vi "Airflow 05.03.16.vi"(0 "Helium":refnum<vi>, 1 "Write refnum In":refnum<file>, 3 "Stop in":refnum<vi>, 5 "Nitrogen":refnum<vi>, 9 "Chemical":refnum<vi>, 11 "Vacuum":refnum<vi>, 12 "Error in":errorcluster, 13 "Boolean":bool, 14 "String out":refnum<vi>) -> (4 "refnum out 2":refnum<file>, 6 "error out":errorcluster, 10 "VISA resource name out":refnum<visa-resource-name>, 15 "Error out VISA":errorcluster)   [LabVIEW 2017]
uses:
  <vilib>/Platform/TimedLoop/XDataNode/timing_clust.ctl
  <vilib>/Platform/TimedLoop/XDataNode/nitl_modes.ctl
  <vilib>/Platform/TimedLoop/XDataNode/wakeup.ctl
  <vilib>/Instr/_visa.llb/VISA Configure Serial Port (Instr).vi
  <vilib>/Utility/file.llb/Read Delimited Spreadsheet (DBL).vi
  <vilib>/platform/TimedLoop/XDataNode/XDataNode.xnode
  <vilib>/Platform/TimedLoop/XDataNode/XDNodeRunTimeDep.lvlib
panel:
  out "Value":dbl
  out "element":dbl
  in  "Vacuum 2":dbl
  out "concatenated string":string
  # "© The Regents of the University of California, Davis campus, 2019. This material is available as open source for research and personal use under a Creative Commons Attribution-NonCommercial-NoDerivatives 4.0 International Public License (https://creativecommons.org/licenses/by-nc-nd/4.0/)."
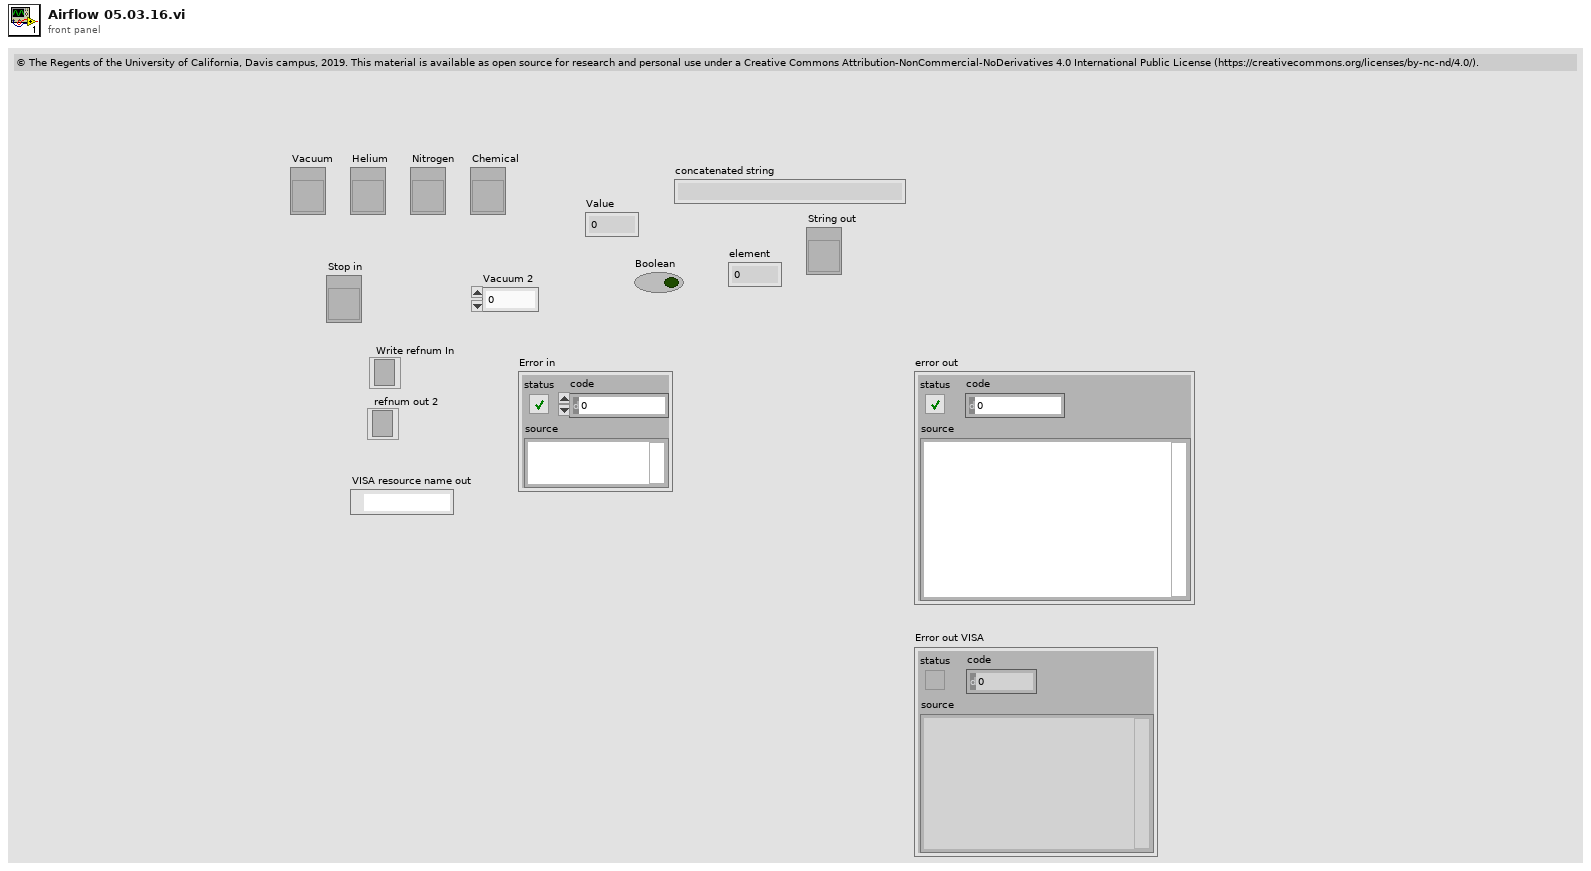
[diagram p1: front panel]
types:
  T1 = typedef "XDNodeRunTimeDep.lvlib/timing_clust.ctl" = cluster{"Expected End [f-1]":u64, "Actual End [f-1]":u64, "Finished Late? [f-1]":bool, "Expected End [i-1]":u64, "Actual End [i-1]":u64, "Finished Late? [i-1]":bool, "Expected Start [i]":u64, "Actual Start [i]":u64, "Expected Start [f]":u64, "Actual Start [f]":u64, "Source Name":string, "Structure Name":string, "Period":i64, "Deadline":i64, "Offset":i64, "Start":i64, "Priority":i32, "Timeout":i32, "Mode":T2, "Wakeup Reason":T3, "Error":errorcluster, "Source Type":string, "Secondary Source Type":string, "Global End Time":u64, "Global Start Time":u64, "Frame Duration":u64, "Iteration Duration":u64, "Assigned CPU":i32, "I/O Scan Engine Mode":u32}
  T2 = typedef "XDNodeRunTimeDep.lvlib/nitl_modes.ctl" = enum32{"No Change", "Process missed periods, maintain original phase", "Discard missed periods, maintain original phase", "Process missed periods, ignore original phase", "Discard missed periods, ignore original phase"}
  T3 = typedef "XDNodeRunTimeDep.lvlib/wakeup.ctl" = enum32{"Normal", "Aborted", "Asynchronous wakeup", "Timing source error", "Timed loop error", "Timeout"}
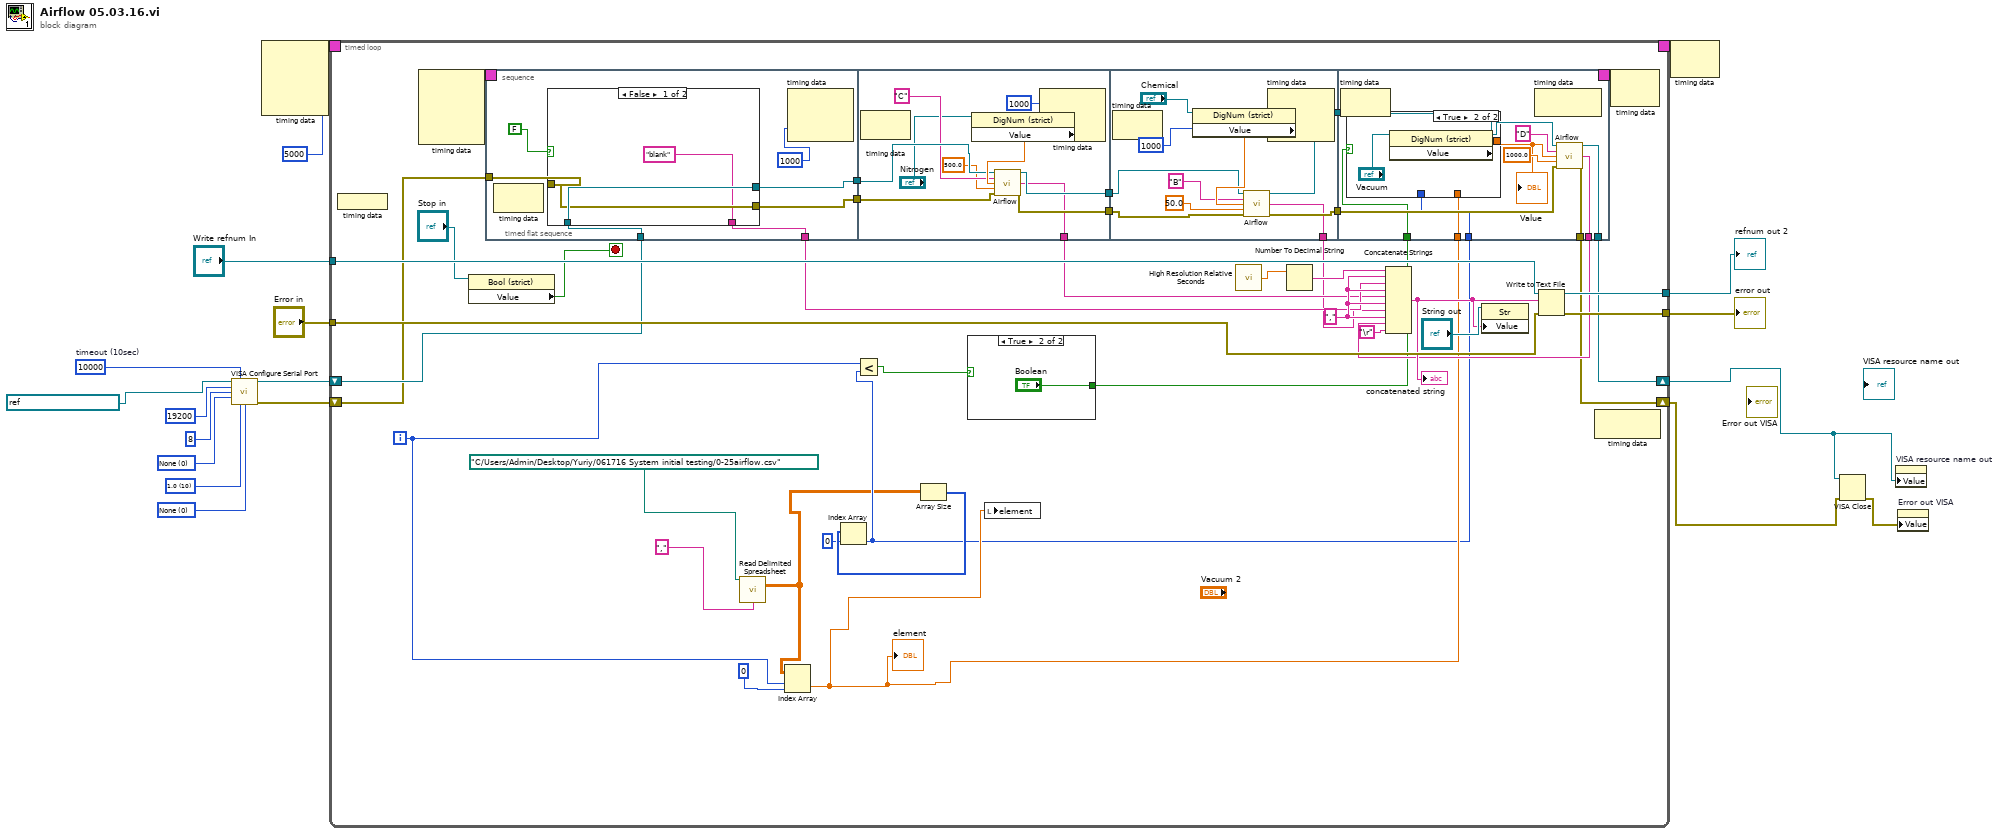
[diagram p0: block diagram]
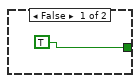
[diagram p2: hidden frame]
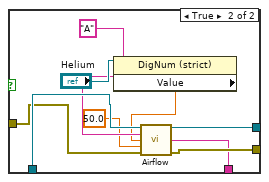
[diagram p3: hidden frame]
diagram:
  w14 = u16 0 items=["None"=0, "XON/XOFF"=1, "RTS/CTS"=2, "DTR/DSR"=4] ("flow control")
  w19 = u16 10 items=["1.0"=10, "1.5"=15, "2.0"=20] ("stop bits")
  w18 = u16 0 items=["None", "Odd", "Even", "Mark", "Space"] ("parity")
  w15 = u32 10000  # timeout (10sec)
  n1 = call-poly "VISA Configure Serial Port"("VISA resource name"=refnum<visa-resource-name> "COM8", "timeout (10sec)"=w15, "baud rate (9600)"=u32 19200 ("baud rate"), "data bits (8)"=u16 8 ("data bits"), "parity (0:none)"=w18, "stop bits (10: 1 bit)"=w19, "flow control (0:none)"=w14) -> ("VISA resource name out"=w13:refnum<visa-resource-name>, "error out"=w12:errorcluster)  [unwired: 7 in]
  n2 = node-c288(i64 5000 ("Period")) -> (w11:T1)  [unwired: 3 in]
  n3 = timed-loop {
    timing: w11 -> [_]
    timing-out: [_] -> w10
    shift-right: [w34] -> w3
    shift-left: w13 -> [w40]
    shift-right: [w33] -> w2
    shift-left: w12 -> [w39]
    tunnel: "Write refnum In" -> [w52]
    tunnel: "Error in" -> [w51]
    tunnel: [w50] -> w8
    tunnel: [w49] -> w5
    i -> [w24]
    stop <- w44 stop-if-true
    w47 = "," ("string")
    n4 = node-c288() -> ()  [unwired: 1 in]
    n5 = node-c288() -> (w32:T1)  [unwired: 4 in]
    n6 = property on="Property Node" class="Bool (strict)"(reference="Stop in") -> ("Value"=w44:bool)  [unwired: 1 in, 2 out]
    n7 = call-poly <vilib>:"Read Delimited Spreadsheet.vi"("file path (dialog if empty)"=path "C:/Users/Admin/Desktop/Yuriy/061716 System initial testing/0-25airflow.csv", "delimiter (\\t)"="," ("delimiter (\\t)")) -> ("all rows"=w21:dbl[][])  [unwired: 8 in, 5 out]
    n8 = Index Array(array=w21, index (row)=w24, index (col)=0 ("disabled index (col)")) -> (element=w25:dbl)
    "element" <- w25
    n9 = Array Size(array=w21) -> (size(s)=w28:i32[])
    n10 = Index Array(array=w28, index=0) -> (element=w23:i32)
    n11 = Less?(x=w24, y=w23) -> (x < y?=w29:bool)
    n12 = case shown="True" w29 {
      tunnel: [TRUE "Boolean"] -> w30
      frame False {
      }
      frame True {
      }
    }
    n13 = timed-sequence {
      timing: w32 -> [_]
      timing-out: [_] -> w31
      tunnel: w40 -> [w71]
      tunnel: w39 -> [w70]
      tunnel: [w69] -> w38
      tunnel: [w66] -> w37
      tunnel: [w63] -> w36
      tunnel: [w60] -> w35
      tunnel: [w59] -> w34
      tunnel: [w58] -> w33
      tunnel: w23 -> [w57]
      tunnel: w30 -> [w56]
      tunnel: w25 -> [w55]
      n14 = timed-flat-sequence {
        tunnel: w71 -> [w78]
        tunnel: w70 -> [w77]
        tunnel: [w76] -> w68
        tunnel: [w75] -> w67
        tunnel: [w74] -> w69
        tunnel: w68 -> [w103]
        tunnel: w67 -> [w102]
        tunnel: [w98] -> w65
        tunnel: [w97] -> w64
        tunnel: [w96] -> w66
        tunnel: w65 -> [w115]
        tunnel: w64 -> [w114]
        tunnel: [w112] -> w62
        tunnel: [w111] -> w61
        tunnel: [w110] -> w63
        tunnel: w62 -> [w131]
        tunnel: w61 -> [w130]
        tunnel: [w129] -> w60
        tunnel: [w128] -> w59
        tunnel: [w127] -> w58
        tunnel: w57 -> [w126]
        tunnel: w56 -> [w125]
        tunnel: w55 -> [w124]
        frame #0 {
          n15 = node-c288() -> ()  [unwired: 1 in, 1 out]
          n16 = case shown="False" FALSE {
            tunnel: w78 -> [w81 w89]
            tunnel: w77 -> [w80 w88]
            tunnel: [w81 w84] -> w76
            tunnel: [w80 w83] -> w75
            tunnel: ["blank" ("delimiter (\\t)") w82] -> w74
            frame False {
            }
            frame True {
              n17 = property on="Property Node" class="DigNum (strict)"(reference="Helium") -> ("Value"=w85:dbl)  [unwired: 1 in, 2 out]
              n18 = call "Airflow.vi"("VISA resource name"=w89, "MFC Control Letter"="A", "Flowrate"=w85, "MFC Max flowrate"=50.0, "error in (no error)"=w88) -> ("VISA resource name 2"=w84:refnum<visa-resource-name>, "substring"=w82:string, "error out"=w83:errorcluster)  [unwired: 8 in]
            }
          }
          n19 = node-c288(i64 1000 ("Start")) -> ()  [unwired: 2 in, 1 out]
        }
        frame #1 {
          n20 = node-c288() -> ()  [unwired: 1 in, 1 out]
          n21 = property on="Property Node" class="DigNum (strict)"(reference="Nitrogen") -> ("Value"=w104:dbl)  [unwired: 1 in, 2 out]
          n22 = call "Airflow.vi"("VISA resource name"=w103, "MFC Control Letter"="C", "Flowrate"=w104, "MFC Max flowrate"=500.0, "error in (no error)"=w102) -> ("VISA resource name 2"=w98:refnum<visa-resource-name>, "substring"=w96:string, "error out"=w97:errorcluster)  [unwired: 8 in]
          n23 = node-c288(i64 1000 ("Start")) -> ()  [unwired: 2 in, 1 out]
        }
        frame #2 {
          n24 = node-c288() -> ()  [unwired: 1 in, 1 out]
          n25 = property on="Property Node" class="DigNum (strict)"(reference="Chemical") -> ("Value"=w118:dbl)  [unwired: 1 in, 2 out]
          n26 = call "Airflow.vi"("VISA resource name"=w115, "MFC Control Letter"="B", "Flowrate"=w118, "MFC Max flowrate"=50.0, "error in (no error)"=w114) -> ("VISA resource name 2"=w112:refnum<visa-resource-name>, "substring"=w110:string, "error out"=w111:errorcluster)  [unwired: 8 in]
          n27 = node-c288(i64 1000 ("Start")) -> ()  [unwired: 2 in, 1 out]
        }
        frame #3 {
          n28 = node-c288() -> ()  [unwired: 1 in, 1 out]
          n29 = case shown="True" w125 {
            tunnel: [w134 w135] -> w123
            tunnel: w126 -> [_ _]
            tunnel: w124 -> [w134 _]
            frame False {
            }
            frame True {
              n30 = property on="Property Node" class="DigNum (strict)"(reference="Vacuum") -> ("Value"=w135:dbl)  [unwired: 1 in, 2 out]
            }
          }
          "Value" <- w123
          n31 = node-c288() -> ()  [unwired: 1 in, 1 out]
          n32 = call "Airflow.vi"("VISA resource name"=w131, "MFC Control Letter"="D", "Flowrate"=w123, "MFC Max flowrate"=1000.0, "error in (no error)"=w130) -> ("VISA resource name 2"=w128:refnum<visa-resource-name>, "substring"=w129:string, "error out"=w127:errorcluster)  [unwired: 8 in]
        }
      }
    }
    n33 = local write "element"(w25) -> ()
    n34 = call <vilib>:"High Resolution Relative Seconds.vi"() -> ("relative seconds"=w48:dbl)
    n35 = Number To Decimal String(number=w48) -> (decimal integer string=w46:string)  [unwired: 1 in]
    n36 = Concatenate Strings(w46, w47, w38, w47, w37, w47, w36, w47, w35, "\r") -> (w41:string)
    "concatenated string" <- w41
    n37 = property on="Property Node" class="Str"(reference="String out", "Value"=w41) -> ()  [unwired: 1 in, 2 out]
    n38 = Write to Text File(file (use dialog)=w52, text=w41, error in=w51) -> (refnum out=w50:refnum<file>, error out=w49:errorcluster)  [unwired: 1 in, 1 out]
    n39 = node-c288() -> ()  [unwired: 1 in, 1 out]
    n40 = node-c288(w31) -> ()  [unwired: 1 out]
  }
  "error out" <- w5
  "refnum out 2" <- w8
  n41 = node-c288(w10) -> ()  [unwired: 1 out]
  n42 = VISA Close(VISA resource name=w3, error in (no error)=w2) -> (error out=w1:errorcluster)
  n43 = property on="VISA resource name out" class="VISAName"("Value"=w3) -> ()  [unwired: 2 in, 2 out]
  n44 = property on="Error out VISA" class="Clust (strict)"("Value"=w1) -> ()  [unwired: 2 in, 2 out]
